vi "Smooth Array.vi"(11 "new element/subarray":dbl) -> (3 "x/y":dbl)   [LabVIEW 2017]
panel:
  in  "dimension size":i32=5
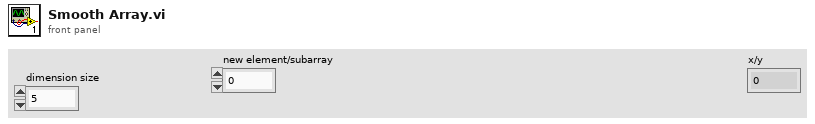
[diagram p1: front panel]
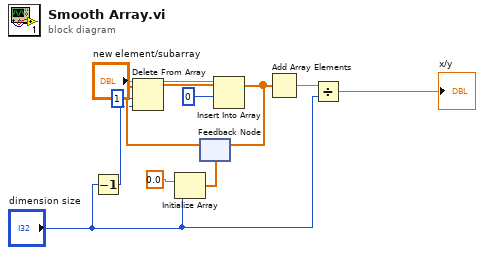
[diagram p0: block diagram]
diagram:
  n1 = Decrement(x="dimension size") -> (x-1=w9:i32)
  n2 = Initialize Array(0.0 ("element"), "dimension size") -> (w11:dbl[])
  n3 = feedback #1(w11) -> (w10:dbl[])
  n4 = Delete From Array(array=w10, length=1, index=w9) -> (array with subset deleted=w7:dbl[])  [unwired: 1 out]
  n5 = Insert Into Array(array=w7, index=0, new element="new element/subarray") -> (w3:dbl[])
  n6 = feedback-in #1(w3) -> ()
  n7 = Add Array Elements(numeric array=w3) -> (sum=w5:dbl)
  n8 = Divide(x=w5, y="dimension size") -> (x/y=→"x/y":dbl)
